vi "ActionVIOnCompile.vi"(8 "error in (no error)":errorcluster, 11 "Device Item Ref in":T1 format="%.0x") -> (0 "error out":errorcluster)   [LabVIEW 2019, in "Software Multi-Plex System Explorer.lvlib"]
uses:
  Software Multi-Plex System Explorer.lvlib
  <vilib>/NI VeriStand/Custom Device API/Custom Device Item Ref.ctl
  Shared/Constants.vi
  <vilib>/NI VeriStand/Custom Device Tools/Custom Device Utility Library/NI VeriStand - Search for All Items by GUID.vi
  <vilib>/NI VeriStand/Custom Device API/Set Item Property (Variant).vi
  <vilib>/NI VeriStand/Custom Device Tools/Custom Device Utility Library/Custom Device Utility Library.lvlib
  <vilib>/NI VeriStand/Custom Device API/Custom Device API.lvlib
  <vilib>/NI/NIVS Inline Async API/_Data Access System Explorer/Data Access System Explorer.lvlib
  Shared/Software Multi-Plex Shared.lvlib
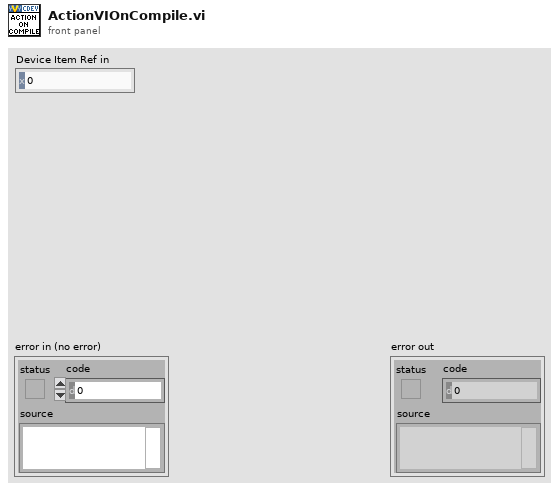
[diagram p1: front panel]
types:
  T1 = typedef "Custom Device API.lvlib/Custom Device Item Ref.ctl" = u64
  T2 = cluster{"Name":string, "Type":enum16{"Output/Write", "Input/Read", "Input/ReadWrite"}, "VS Refs":T1[]}
  T3 = enum16{"Output/Write", "Input/Read", "Input/ReadWrite"}
  T4 = typedef "Custom Device API.lvlib/Custom Device Item Info.ctl" = cluster{"Name":string, "Is Channel":bool, "GUID":string, "Is Waveform":bool}
  T5 = cluster{"Name":string, "Type":enum16{"Output/Write", "Input/Read", "Input/ReadWrite"}, "VS Refs":T1[]}[]
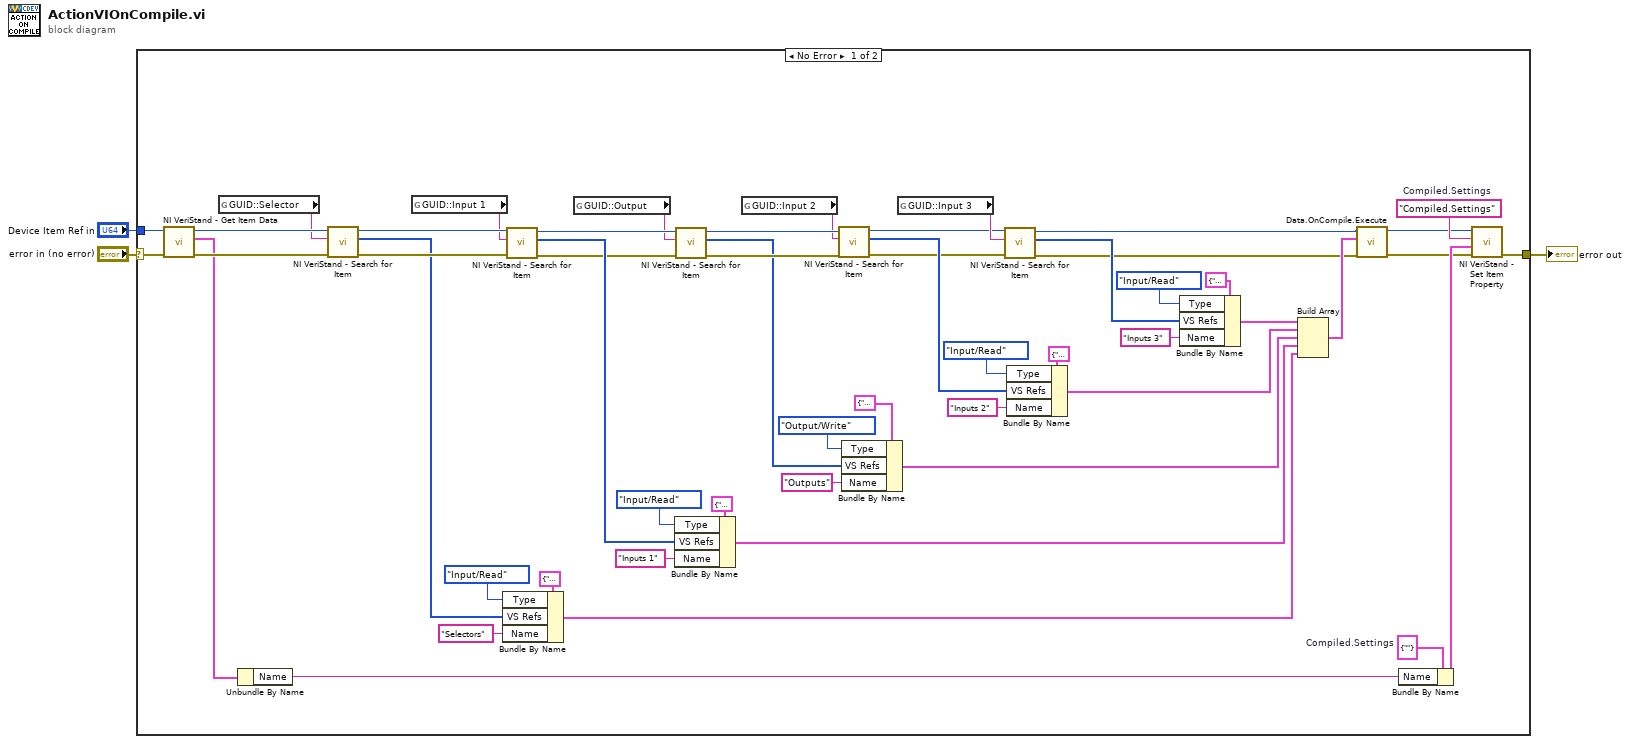
[diagram p0: block diagram]
diagram:
  n1 = case shown="No Error" "error in (no error)" {
    selector: "error in (no error)" -> [w53 w57]
    tunnel: [w54 w57] -> w2
    tunnel: "Device Item Ref in" -> [w52 _]
    frame No Error {
      w42 = cluster{"Name":string} {"Name"=""}  # Compiled.Settings
      w56 = "Compiled.Settings"  # Compiled.Settings
      n2 = call <vilib>:"NI VeriStand - Get Item Data.vi"("error in (no error)"=w53, "Item Ref in"=w52) -> ("error out"=w50:errorcluster, "Item Info"=w49:T4, "Item Ref out"=w51:T1)  [unwired: 6 in, 1 out]
      n3 = global read "Constants.vi" "GUID::Selector"() -> (w41:string)
      n4 = Unbundle By Name(w49) -> ("Name"=w48:string)
      n5 = call-poly <vilib>:"NI VeriStand - Search for Item.vi"("error in"=w50, "Item GUID"=w41, "Section Ref in"=w51) -> ("error out"=w40:errorcluster, "Item Refs"=w36:T1[], "Section Ref out"=w39:T1)  [unwired: 5 in, 1 out]
      n6 = global read "Constants.vi" "GUID::Input 1"() -> (w38:string)
      n7 = Bundle By Name(cluster=T2 {"Name"="", "Type"=enum."Output/Write", "VS Refs"=[]} ("Group"), "Type"=T3."Input/Read", "VS Refs"=w36, "Name"="Selectors") -> (w24:T2)
      n8 = call-poly <vilib>:"NI VeriStand - Search for Item.vi"("error in"=w40, "Item GUID"=w38, "Section Ref in"=w39) -> ("error out"=w22:errorcluster, "Item Refs"=w32:T1[], "Section Ref out"=w21:T1)  [unwired: 5 in, 1 out]
      n9 = global read "Constants.vi" "GUID::Output"() -> (w20:string)
      n10 = Bundle By Name(cluster=T2 {"Name"="", "Type"=enum."Output/Write", "VS Refs"=[]} ("Group"), "Type"=T3."Input/Read", "VS Refs"=w32, "Name"="Inputs 1") -> (w25:T2)
      n11 = call-poly <vilib>:"NI VeriStand - Search for Item.vi"("error in"=w22, "Item GUID"=w20, "Section Ref in"=w21) -> ("error out"=w19:errorcluster, "Item Refs"=w17:T1[], "Section Ref out"=w18:T1)  [unwired: 5 in, 1 out]
      n12 = global read "Constants.vi" "GUID::Input 2"() -> (w16:string)
      n13 = call-poly <vilib>:"NI VeriStand - Search for Item.vi"("error in"=w19, "Item GUID"=w16, "Section Ref in"=w18) -> ("error out"=w8:errorcluster, "Item Refs"=w15:T1[], "Section Ref out"=w9:T1)  [unwired: 5 in, 1 out]
      n14 = Bundle By Name(cluster=T2 {"Name"="", "Type"=enum."Output/Write", "VS Refs"=[]} ("Group"), "Type"=T3."Output/Write", "VS Refs"=w17, "Name"="Outputs") -> (w26:T2)
      n15 = global read "Constants.vi" "GUID::Input 3"() -> (w11:string)
      n16 = call-poly <vilib>:"NI VeriStand - Search for Item.vi"("error in"=w8, "Item GUID"=w11, "Section Ref in"=w9) -> ("error out"=w7:errorcluster, "Item Refs"=w10:T1[], "Section Ref out"=w6:T1)  [unwired: 5 in, 1 out]
      n17 = Bundle By Name(cluster=T2 {"Name"="", "Type"=enum."Output/Write", "VS Refs"=[]} ("Group"), "Type"=T3."Input/Read", "VS Refs"=w15, "Name"="Inputs 2") -> (w27:T2)
      n18 = Bundle By Name(cluster=T2 {"Name"="", "Type"=enum."Output/Write", "VS Refs"=[]} ("Group"), "Type"=T3."Input/Read", "VS Refs"=w10, "Name"="Inputs 3") -> (w4:T2)
      n19 = Build Array(w4, w27, w26, w25, w24) -> (w23:T5)
      n20 = call <vilib>:"Data.OnCompile.Execute.vi"("error in"=w7, "VS Ref Groups"=w23, "Custom Device Ref"=w6) -> ("error out"=w43:errorcluster, "Custom Device Ref"=w5:T1)  [unwired: 7 in]
      n21 = Bundle By Name(cluster=w42, "Name"=w48) -> (w55:cluster{"Name":string})
      n22 = call-poly <vilib>:"NI VeriStand - Set Item Property.vi"("error in (no error)"=w43, "Value"=w55, "Property Name"=w56, "Item Ref in"=w5) -> ("error out"=w54:errorcluster)  [unwired: 5 in, 2 out]
    }
    frame Error {
    }
  }
  "error out" <- w2
